vi "FastMap - Read Row.vi"(10 "Row":i32, 11 "fast map in":refnum<data-value>) -> (2 "square states":T1[](array[typedef]), 3 "fast map out":refnum<data-value>)   [LabVIEW 2015, in "DS Square.lvlib"]
uses:
  DS Square.lvlib
  Square State Fast.ctl
  Fast Map.ctl
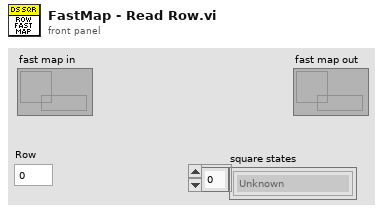
[diagram p1: front panel]
types:
  T1 = typedef "DS Square.lvlib/Square State Fast.ctl" = enum8{"Unknown", "Empty", "Occupied - Active", "Occupied - Cool Down", "Attacked", "Enemy", "Enemy Wall"}
  T2 = typedef "DS Square.lvlib/Fast Map.ctl" = cluster{"state":T1[][], "updated":i32[][]}
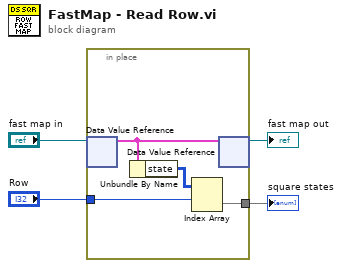
[diagram p0: block diagram]
diagram:
  n1 = in-place {
    in-place-border: "Row" -> [w6]
    in-place-border: [w5] -> w1
    n2 = in-place-dvr #1("fast map in") -> (w8:T2)  [unwired: 1 out]
    n3 = Unbundle By Name(w8) -> ("state"=w7:T1[][])
    n4 = Index Array(array=w7, index (row)=w6) -> (element=w5:T1[])  [unwired: 1 in]
    n5 = in-place-dvr #1(w8) -> (→"fast map out":refnum<data-value>)  [unwired: 1 out]
  }
  "square states" <- w1
